vi "qSPV.vi"(0 "System no.":i32=1 min=1 max=4 step=1, 1 "Memory Type":T2, 2 "ContainerUnit":string, 3 "FunctionUnit":string, 4 "ParameterID":string, 5 "error in":errorcluster) -> (14 "Parameters":T1[](array[typedef]), 19 "error out":errorcluster)   [LabVIEW 2026]
doc: "Reads parameter list from the memories of the controller. \nDepending on the argument(s) used, the query is limited to a specific memory type and parameters."
uses:
  MemoryType.ctl
  Parameter Set.ctl
  <vilib>/Utility/error.llb/Trim Whitespace One-Sided.vi
panel:
  # "Returns parameter value(s) for queried Memory, ContainerUnit, FunctionUnit and ParameterID. The order is as described. E.g. to get the parameters for a specific FunctionUnit you have to define the MemoryType and ContainerUnit for it"
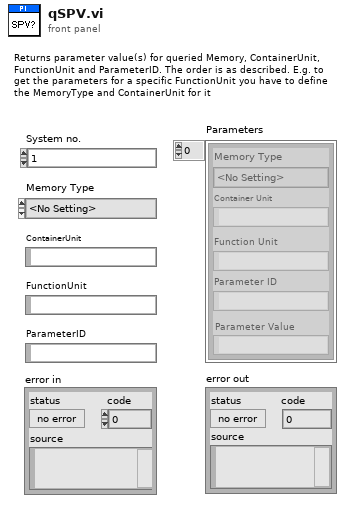
[diagram p1: front panel]
types:
  T1 = typedef "Parameter Set.ctl" = cluster{"Memory Type":T2, "Container Unit":string, "Function Unit":string, "Parameter ID":string, "Parameter Value":string}
  T2 = typedef "MemoryType.ctl" = enum16{"<No Setting>", "RAM", "FLASH", "TMP"}
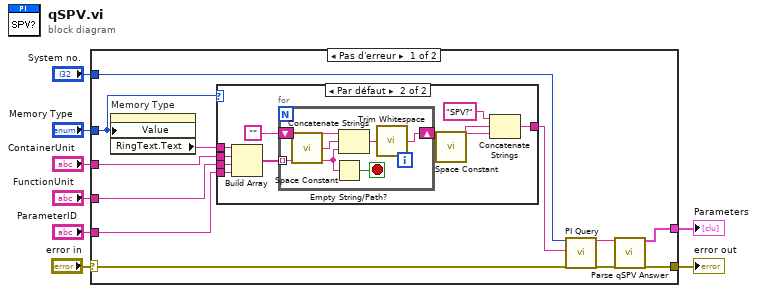
[diagram p0: block diagram]
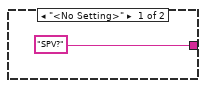
[diagram p2: hidden frame]
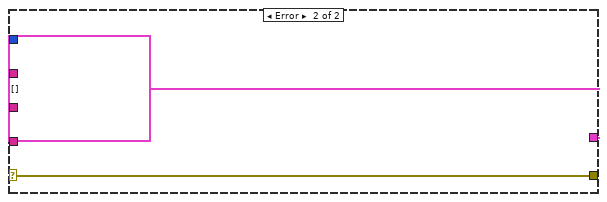
[diagram p3: hidden frame]
diagram:
  n1 = case shown="Pas d'erreur" "error in" {
    selector: "error in" -> [w15 w39]
    tunnel: "System no." -> [w13 _]
    tunnel: [w10 w39] -> w7
    tunnel: "Memory Type" -> [w16 _]
    tunnel: "ContainerUnit" -> [w19 _]
    tunnel: "FunctionUnit" -> [w18 _]
    tunnel: "ParameterID" -> [w17 _]
    tunnel: [w12 T1[] []] -> w1
    frame No Error {
      n2 = property on="Memory Type" class="Énum (strict)"("Value"=w16) -> ("RingText.Text"=w20:string)  [unwired: 2 in, 2 out]
      n3 = case shown="Par défaut" w16 {
        tunnel: w20 -> [_ w31]
        tunnel: w19 -> [_ w30]
        tunnel: w18 -> [_ w29]
        tunnel: w17 -> [_ w28]
        tunnel: ["SPV?" w25] -> w14
        frame "<No Setting>" {
        }
        frame Default {
          n4 = Build Array(w31, w30, w29, w28) -> (w22:string[])
          n5 = for {
            tunnel: w22 -> [w34] mode=indexing
            shift-right: [w36] -> w26
            shift-left: "" ("trimmed string") -> [w37]
            stop <- w32 stop-if-true
            n6 = call <vilib>:"Space Constant.vi"() -> ("String"=w35:string)
            n7 = Empty String/Path?(string/path=w34) -> (empty?=w32:bool)
            n8 = Concatenate Strings(w37, w35, w34) -> (w33:string)
            n9 = call <vilib>:"Trim Whitespace.vi"("string"=w33) -> ("trimmed string"=w36:string)  [unwired: 1 in]
          }
          n10 = call <vilib>:"Space Constant.vi"() -> ("String"=w24:string)
          n11 = Concatenate Strings("SPV?", w24, w26) -> (w25:string)
        }
      }
      n12 = call "PI Query.vi"("System no."=w13, "String to send"=w14, "error in"=w15) -> ("String read"=w11:string, "error out"=w9:errorcluster)  [unwired: 13 in, 2 out]
      n13 = call "Parse qSPV Answer.vi"("Answer To Parse"=w11, "error in"=w9) -> ("Array of Parameters"=w12:T1[], "error out"=w10:errorcluster)  [unwired: 16 in]
    }
    frame Error {
    }
  }
  "error out" <- w7
  "Parameters" <- w1
